vi "Write Error .vi"(10 "Error":T1, 11 "STEP in":refnum<class "STEP.lvclass">) -> (3 "STEP out":refnum<class "STEP.lvclass">)   [LabVIEW 2014, in "SeqLoop.lvlib" / "STEP Classes.lvlib" / "STEP.lvclass"]
uses:
  STEP.lvclass
  TypeDefs/LogicParsedExpression.ctl
  STEP.lvclass/STEP.ctl
  SeqLoop.lvlib
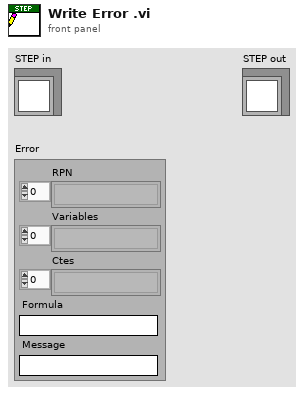
[diagram p1: front panel]
types:
  T1 = typedef "SeqLoop.lvlib/LogicParsedExpression.ctl" = cluster{"RPN ":string[], "Variables":string[], "Ctes":string[], "Formula":string, "Message":string}
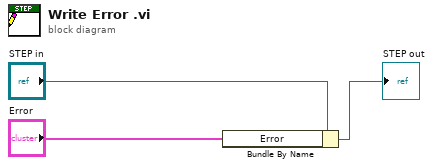
[diagram p0: block diagram]
diagram:
  n1 = Bundle By Name(cluster="STEP in", "Error"="Error") -> (→"STEP out":refnum<class "STEP.lvclass">)
